vi "SHA-256 File Checksum.vi"(8 "error in":errorcluster, 11 "path":path) -> (0 "error out":errorcluster, 3 "digest":string)   [LabVIEW 2020, in "NI_Message Digest API.lvlib"]
doc: "Computes the message digest on the contents of a file. You must manually select the polymorphic instance you want to use."
uses:
  <vilib>/security/Message Digest/API/NI_Message Digest API.lvlib
  07e2d62d-d65e-48d1-912a-6d9031207283.vi
  07e2d62d-d65e-48d1-912a-6d9031207283.vi/500e482c-8ac5-3fe1-005b-a2c31de3883f.vi
  <vilib>/security/Message Digest/SHA-2/SHA-256/Get Block Size.vi
  <vilib>/security/Message Digest/SHA-2/SHA-256/Reset.vi
  <vilib>/security/Message Digest/SHA-2/SHA-256/Append Block.vi
  <vilib>/security/Message Digest/SHA-2/SHA-256/Pad.vi
  <vilib>/security/Message Digest/SHA-2/SHA-256/Get Digest.vi
  <vilib>/security/Message Digest/SHA-2/SHA-256/NI_SHA-256.lvclass
  <vilib>/Bit Manipulation/NI_Bit Manipulation.lvlib
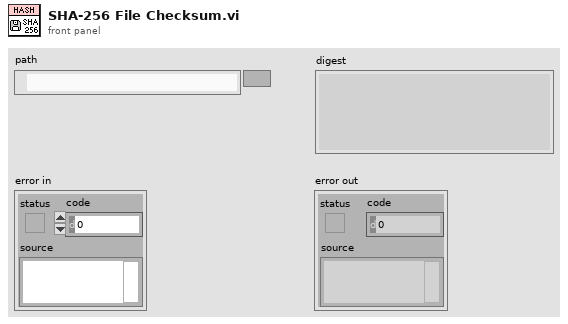
[diagram p1: front panel]
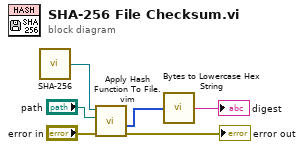
[diagram p0: block diagram]
diagram:
  n1 = call <vilib>:"SHA-256.vi"() -> ("Hash Function out"=w2:refnum<class "NI_SHA-256.lvclass">)
  n2 = call "Apply Hash Function To File.vim"("error in"="error in", "path"="path", "Hash Function in (SHA-256)"=w2) -> ("error out"=→"error out":errorcluster, "digest"=w1:u8[])  [unwired: 6 in, 1 out]
  n3 = call <vilib>:"Bytes to Lowercase Hex String.vi"("bytes"=w1) -> ("hex string"=→"digest":string)
